vi "Disable Controls.vi"(7 "Disabled":T1(ring), 8 "error in (no error)":errorcluster, 11 "Array":refnum<vi>[](array[refnum])) -> (0 "error out":errorcluster)   [LabVIEW 2017, in "Shared Variables CD 2.0 Configuration.lvlib"]
uses:
  Shared Variables CD 2.0 Configuration.lvlib
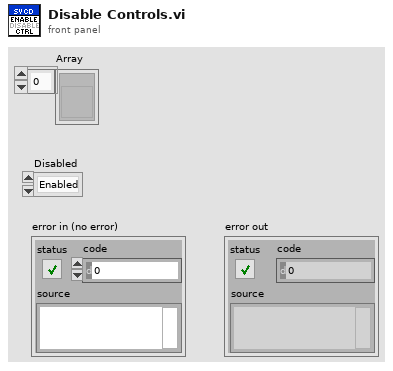
[diagram p1: front panel]
types:
  T1 = enum8{"Enabled", "Disabled", "Disabled and Grayed Out"}
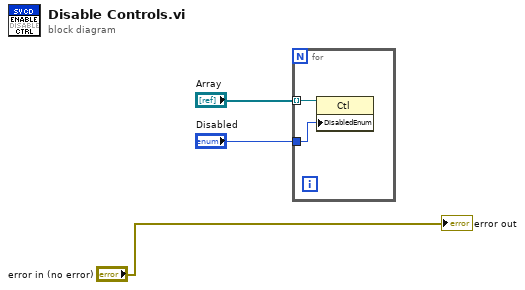
[diagram p0: block diagram]
diagram:
  n1 = for {
    tunnel: "Disabled" -> [w5]
    tunnel: "Array" -> [w4] mode=indexing
    n2 = property on="Property Node" class="Ctl"(reference=w4, "DisabledEnum"=w5) -> ()  [unwired: 1 in, 2 out]
  }
  "error out" <- "error in (no error)"
